vi "探头滤波次数.vi"(7 "校准参数":u16(ring) caption="校准参数：" items=["pH", "DO", "浊度", "电导率", "叶绿素a", "藻密度", "ORP", "DO2"], 8 "error in (no error)":errorcluster caption="错误输入（无错误）", 11 "滤波次数":sgl) -> (0 "error out":errorcluster caption="错误输出")   [LabVIEW 2016, in "斯坦道多参数.lvlib"]
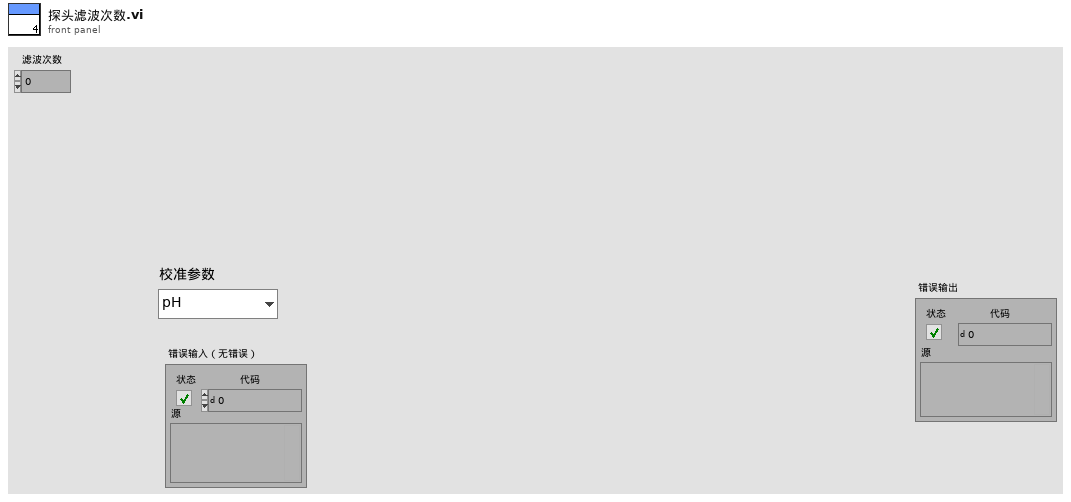
[diagram p1: front panel]
types:
  T1 = enum16{"NULL", "pH", "Cond", "DO", "Turb", "ORP"}
  T2 = cluster{"pH":u32, "DO":u32, "Cond":u32, "Turb":u32, "叶绿素a":u32, "藻密度":u32, "ORP":u32, "COD":u32}
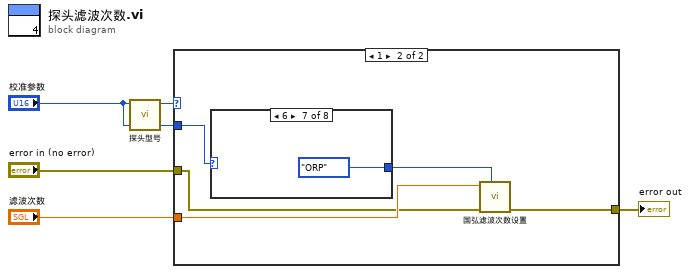
[diagram p0: block diagram]
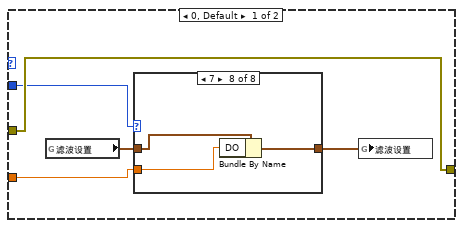
[diagram p2: hidden frame]
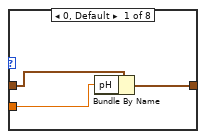
[diagram p3: hidden frame]
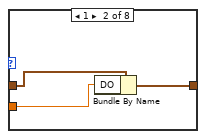
[diagram p4: hidden frame]
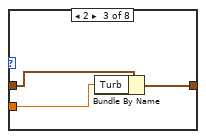
[diagram p5: hidden frame]
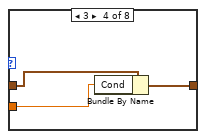
[diagram p6: hidden frame]
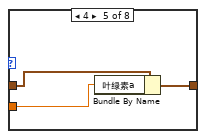
[diagram p7: hidden frame]
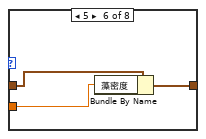
[diagram p8: hidden frame]
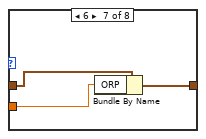
[diagram p9: hidden frame]
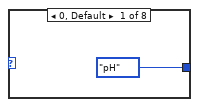
[diagram p10: hidden frame]
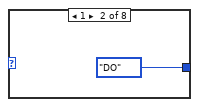
[diagram p11: hidden frame]
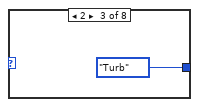
[diagram p12: hidden frame]
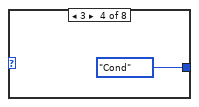
[diagram p13: hidden frame]
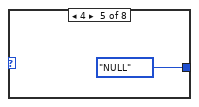
[diagram p14: hidden frame]
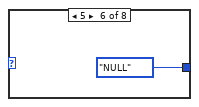
[diagram p15: hidden frame]
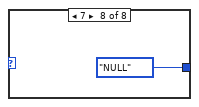
[diagram p16: hidden frame]
diagram:
  n1 = call "探头型号.vi"("校准参数"="校准参数") -> ("探头型号"=w5:u16)  [unwired: 8 in, 2 out]
  n2 = case shown="1" w5 {
    tunnel: "校准参数" -> [w7 w39]
    tunnel: "error in (no error)" -> [w10 w36]
    tunnel: [w10 w35] -> w2
    tunnel: "滤波次数" -> [w6 w37]
    frame 0, Default {
      n3 = global read "断电保存变量.vi" "滤波设置"() -> (w9:T2)
      n4 = case shown="7" w7 {
        tunnel: w6 -> [w11 w15 w17 w20 w23 w26 w29 w32]
        tunnel: w9 -> [w13 w16 w19 w22 w24 w27 w31 w33]
        tunnel: [w12 w14 w18 w21 w25 w28 w30 w34] -> w8
        frame 0, Default {
          n5 = Bundle By Name(cluster=w13, "pH"=w11) -> (w12:T2)
        }
        frame 1 {
          n6 = Bundle By Name(cluster=w16, "DO"=w15) -> (w14:T2)
        }
        frame 2 {
          n7 = Bundle By Name(cluster=w19, "Turb"=w17) -> (w18:T2)
        }
        frame 3 {
          n8 = Bundle By Name(cluster=w22, "Cond"=w20) -> (w21:T2)
        }
        frame 4 {
          n9 = Bundle By Name(cluster=w24, "叶绿素a"=w23) -> (w25:T2)
        }
        frame 5 {
          n10 = Bundle By Name(cluster=w27, "藻密度"=w26) -> (w28:T2)
        }
        frame 6 {
          n11 = Bundle By Name(cluster=w31, "ORP"=w29) -> (w30:T2)
        }
        frame 7 {
          n12 = Bundle By Name(cluster=w33, "DO"=w32) -> (w34:T2)
        }
      }
      n13 = global write "断电保存变量.vi" "滤波设置"(w8) -> ()
    }
    frame 1 {
      n14 = case shown="6" w39 {
        tunnel: [T1."pH" ("探头") T1."DO" ("探头") T1."Turb" ("探头") T1."Cond" ("探头") T1."NULL" ("探头") T1."NULL" ("探头") T1."ORP" ("探头") T1."NULL" ("探头")] -> w38
        frame 0, Default {
        }
        frame 1 {
        }
        frame 2 {
        }
        frame 3 {
        }
        frame 4 {
        }
        frame 5 {
        }
        frame 6 {
        }
        frame 7 {
        }
      }
      n15 = call "国弘滤波次数设置.vi"("探头"=w38, "error in (no error)"=w36, "滤波次数"=w37) -> ("error out"=w35:errorcluster)  [unwired: 7 in, 1 out]
    }
  }
  "error out" <- w2
